vi "Inverse DST.vi"   [LabVIEW 2024, in "NI_AALPro.lvlib"]
doc: "<p>Computes the inverse Discrete Sine Transform (DST) of the input sequence <strong>DST {X}</strong>. Wire data to the <strong>DST {X}</strong> input to determine the polymorphic instance to use or <a href=\"nihelplauncher://docs/csh?context=lvcore_lvhowto_selectingdefaultinstpolyvi\">manually select</a> the instance.\n</p>"
uses:
  NI_AALPro.lvlib
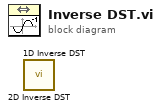
[diagram p0: block diagram]
diagram:
  n1 = call "2D Inverse DST.vi"() -> ()  [unwired: 10 in, 2 out]
  n2 = call "1D Inverse DST.vi"() -> ()  [unwired: 10 in, 2 out]
